vi "Save PID Configuration.vi"(8 "Error In":errorcluster, 10 "SP":dbl=0.55, 11 "PID Parameters":cluster{"Kp":dbl, "Ti [s]":dbl, "Td [s]":dbl}={"Kp"=0.55, "Ti [s]"=18.0, "Td [s]"=0.0}) -> (0 "Error Out":errorcluster)   [LabVIEW 2018]
uses:
  <vilib>/Utility/config.llb/Write Key (Double).vi
  <vilib>/Utility/config.llb/NI_LVConfig.lvlib
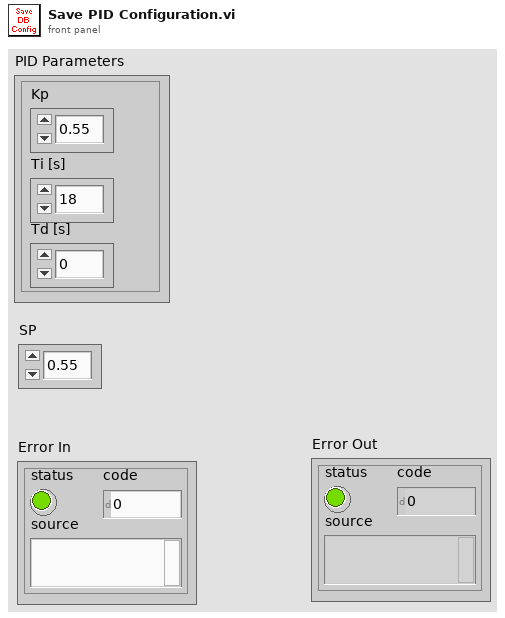
[diagram p1: front panel]
types:
  T1 = typedef "NI_LVConfig.lvlib/Config Data RefNum.ctl" = refnum<k1>
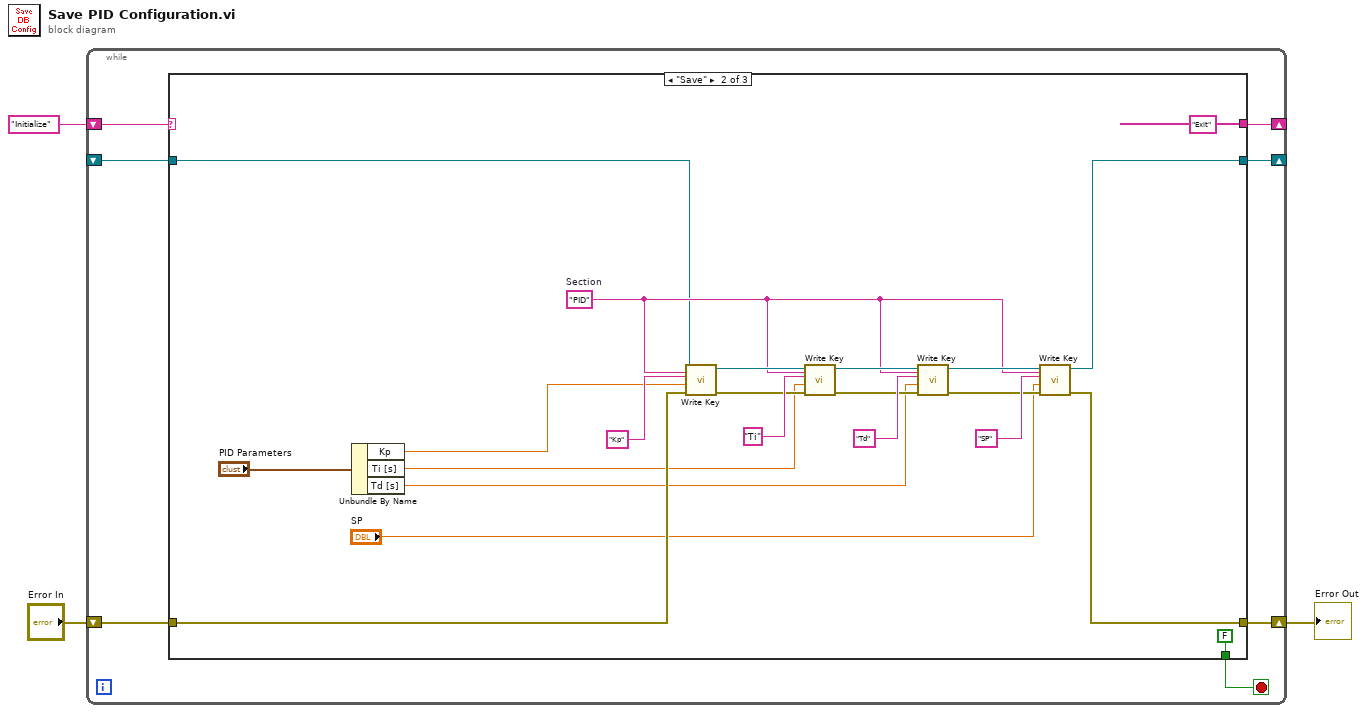
[diagram p0: block diagram]
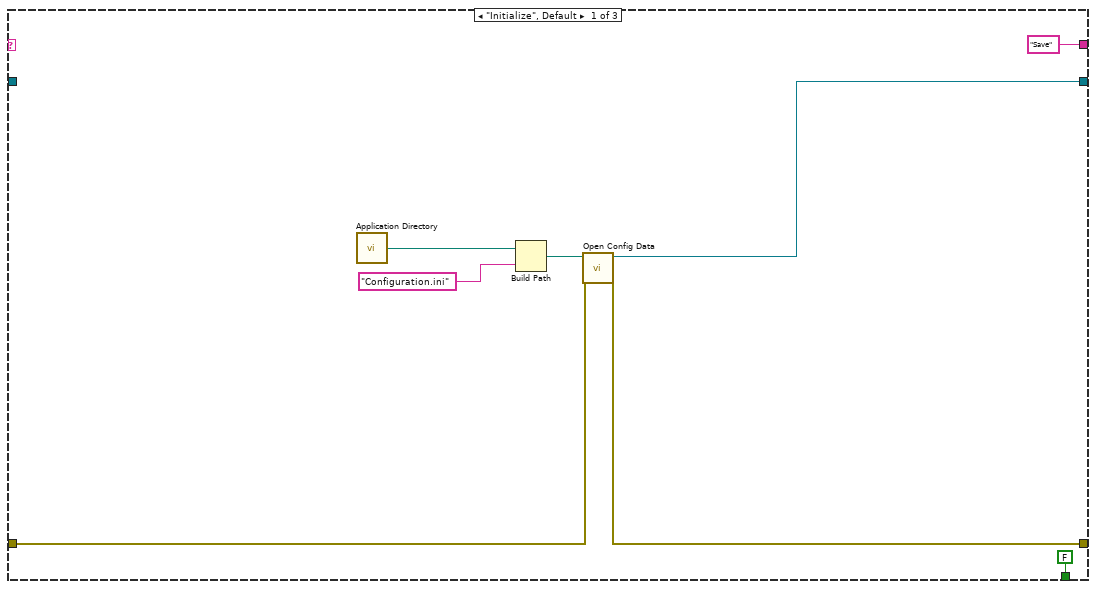
[diagram p2: hidden frame]
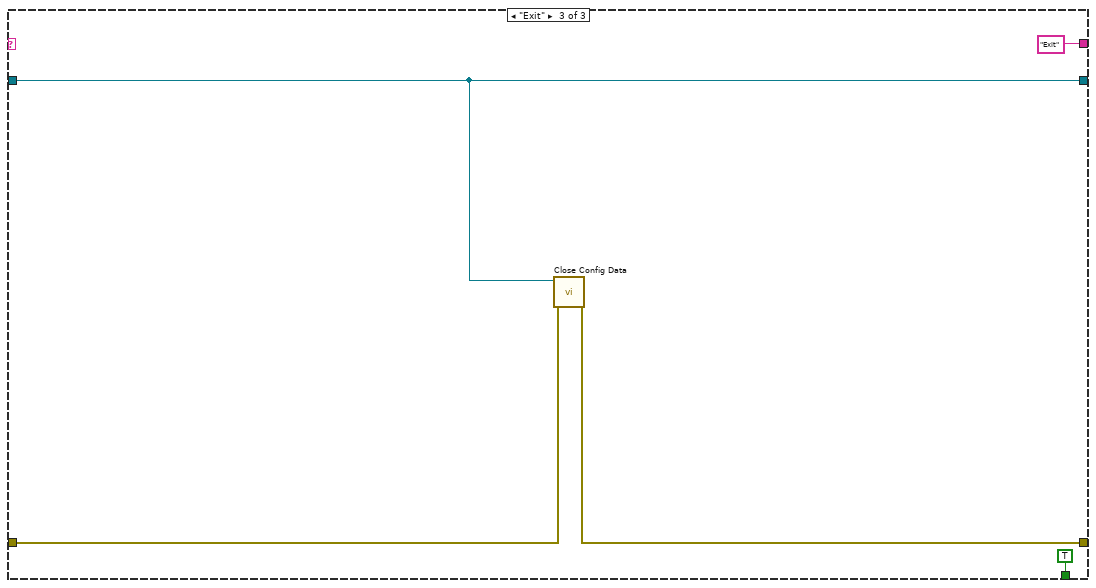
[diagram p3: hidden frame]
diagram:
  n1 = while {
    shift-right: [w6] -> _
    shift-left: "Initialize" ("key") -> [w10]
    shift-right: [w7] -> _
    shift-left: _ -> [w9]
    shift-right: [w4] -> w1
    shift-left: "Error In" -> [w8]
    stop <- w5 stop-if-true
    n2 = case shown="\"Save\"" w10 {
      tunnel: w9 -> [_ w25 w43]
      tunnel: w8 -> [w12 w27 w42]
      tunnel: [w13 w24 w43] -> w7
      tunnel: ["Save" ("key") "Exit" ("key") "Exit" ("key")] -> w6
      tunnel: [FALSE FALSE TRUE] -> w5
      tunnel: [w11 w26 w41] -> w4
      frame "Initialize", Default {
        n3 = call <vilib>:"Application Directory.vi"() -> ("Application Directory"=w16:path)
        n4 = Build Path(base path=w16, name or relative path="Configuration.ini") -> (appended path=w14:path)
        n5 = call <vilib>:"Open Config Data.vi"("error in (no error)"=w12, "configuration file path"=w14) -> ("error out"=w11:errorcluster, "refnum"=w13:T1)  [unwired: 7 in, 1 out]
      }
      frame "Save" {
        w28 = "PID"  # Section
        n6 = Unbundle By Name("PID Parameters") -> ("Kp"=w23:dbl, "Ti [s]"=w22:dbl, "Td [s]"=w21:dbl)
        n7 = call-poly <vilib>:"Write Key.vi"("section"=w28, "error in (no error)"=w27, "value"=w23, "key"="Kp", "refnum"=w25) -> ("error out"=w37:errorcluster, "refnum out"=w36:T1)  [unwired: 4 in, 1 out]
        n8 = call-poly <vilib>:"Write Key.vi"("section"=w28, "error in (no error)"=w37, "value"=w22, "key"="Ti", "refnum"=w36) -> ("error out"=w31:errorcluster, "refnum out"=w32:T1)  [unwired: 4 in, 1 out]
        n9 = call-poly <vilib>:"Write Key.vi"("section"=w28, "error in (no error)"=w31, "value"=w21, "key"="Td", "refnum"=w32) -> ("error out"=w29:errorcluster, "refnum out"=w30:T1)  [unwired: 4 in, 1 out]
        n10 = call-poly <vilib>:"Write Key.vi"("section"=w28, "error in (no error)"=w29, "value"="SP", "key"="SP", "refnum"=w30) -> ("error out"=w26:errorcluster, "refnum out"=w24:T1)  [unwired: 4 in, 1 out]
      }
      frame "Exit" {
        n11 = call <vilib>:"Close Config Data.vi"("error in (no error)"=w42, "refnum"=w43) -> ("error out"=w41:errorcluster)  [unwired: 8 in, 1 out]
      }
    }
  }
  "Error Out" <- w1
